vi "load.vi"(8 "error in (no error)":errorcluster, 10 "Node":refnum<k20>, 11 "HP83623A_RF_Generator in":refnum<class "HP83623A_RF_Generator.lvclass">) -> (0 "error out":errorcluster, 2 "node out":refnum<k20>, 3 "HP83623A_RF_Generator out":refnum<class "HP83623A_RF_Generator.lvclass">)   [LabVIEW 2013, in "HP83623A_RF_Generator.lvclass"]
uses:
  HP83623A_RF_Generator.lvclass
  HP83623A.ctl
  HP83623A_RF_Generator.lvclass/HP83623A_RF_Generator.ctl
  <vilib>/xml/Close Reference(Node).vi
  <vilib>/xml/NI_XML.lvlib
  <resource>/objmgr/DOMUserDefRef.rc
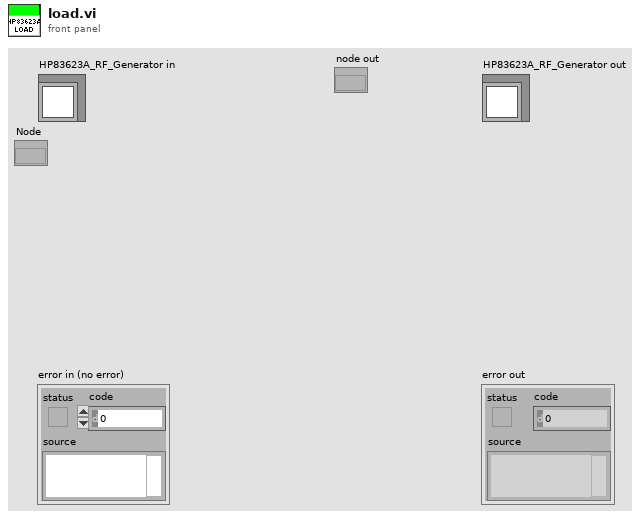
[diagram p1: front panel]
types:
  T1 = typedef "HP83623A_RF_Generator.lvclass/HP83623A.ctl" = cluster{"Frequency (Hz)":dbl, "Power (dBm)":dbl, "Enabled":bool, "initialized":bool, "RF Output On/Off":bool, "External Trigger?":bool, "VISA Session":refnum<visa-resource-name>, "Generator Name":string}
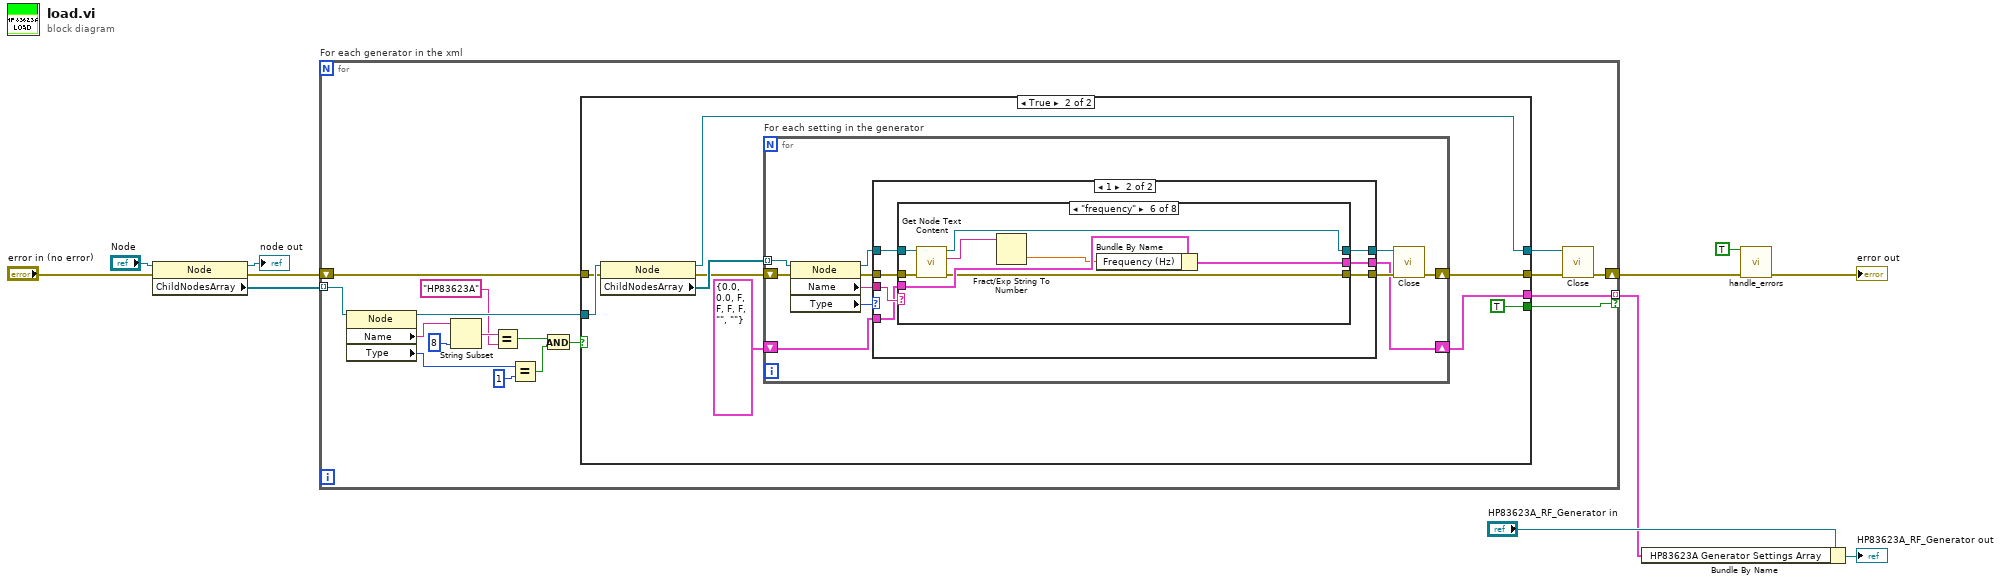
[diagram p0: block diagram]
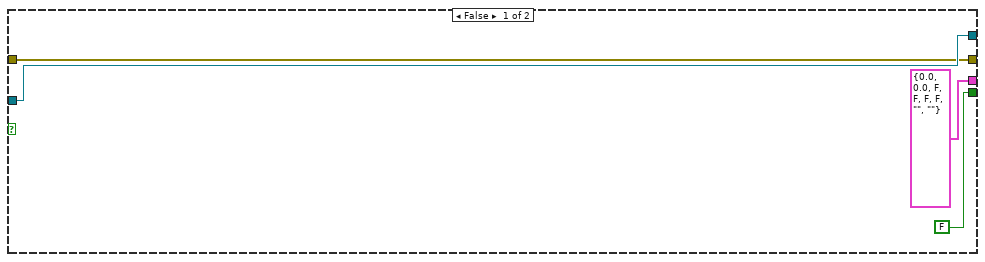
[diagram p2: hidden frame]
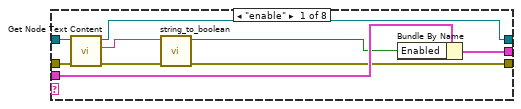
[diagram p4: hidden frame]
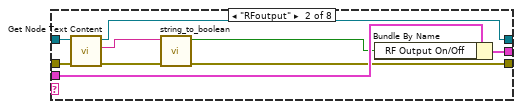
[diagram p5: hidden frame]
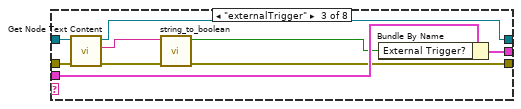
[diagram p6: hidden frame]
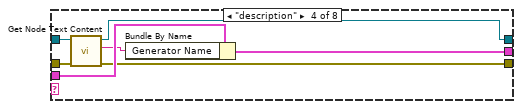
[diagram p7: hidden frame]
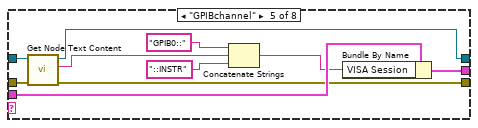
[diagram p8: hidden frame]
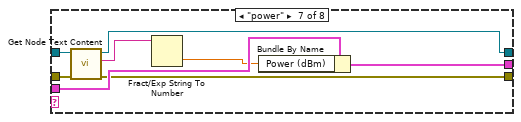
[diagram p9: hidden frame]
diagram:
  n1 = property class="Node"(reference="Node", error in="error in (no error)") -> (reference out=→"node out":refnum<k20>, error out=w4:errorcluster, "ChildNodesArray"=w5:refnum<k20>[])
  n2 = for "For each generator in the xml" {
    tunnel: w5 -> [w23] mode=indexing
    shift-right: [w25] -> w3
    shift-left: w4 -> [w28]
    tunnel: [w12] -> w9 mode=indexing if=w24
    n3 = property class="Node"(reference=w23) -> (reference out=w22:refnum<k20>, "Name"=w18:string, "Type"=w21:i32)  [unwired: 1 in, 1 out]
    n4 = String Subset(string=w18, length (rest)=8 ("length (rest)")) -> (substring=w16:string)  [unwired: 1 in]
    n5 = Equal?(x=w16, y="HP83623A") -> (x = y?=w14:bool)
    n6 = Equal?(x=w21, y=1) -> (x = y?=w19:bool)
    n7 = And(x=w14, y=w19) -> (x .and. y?=w13:bool)
    n8 = case shown="True" w13 {
      tunnel: w22 -> [w32 w41]
      tunnel: w28 -> [w31 w40]
      tunnel: [w32 w37] -> w27
      tunnel: [w31 w36] -> w26
      tunnel: [T1 {"Frequency (Hz)"=0.0, "Power (dBm)"=0.0, "Enabled"=FALSE, "initialized"=FALSE, "RF Output On/Off"=FALSE, "External Trigger?"=FALSE, "VISA Session"="", "Generator Name"=""} ("hp83623a Settings In") w35] -> w12
      tunnel: [FALSE TRUE] -> w24
      frame False {
      }
      frame True {
        n9 = property class="Node"(reference=w41, error in=w40) -> (reference out=w37:refnum<k20>, error out=w38:errorcluster, "ChildNodesArray"=w39:refnum<k20>[])
        n10 = for "For each setting in the generator" {
          shift-right: [w45] -> w36
          shift-left: w38 -> [w49]
          tunnel: w39 -> [w52] mode=indexing
          shift-right: [w43] -> w35
          shift-left: T1 {"Frequency (Hz)"=0.0, "Power (dBm)"=0.0, "Enabled"=FALSE, "initialized"=FALSE, "RF Output On/Off"=FALSE, "External Trigger?"=FALSE, "VISA Session"="", "Generator Name"=""} ("hp83623a Settings In") -> [w44]
          n11 = property class="Node"(reference=w52, error in=w49) -> (reference out=w47:refnum<k20>, error out=w50:errorcluster, "Name"=w51:string, "Type"=w42:i32)
          n12 = case shown="1" w42 {
            tunnel: w51 -> [_ w62]
            tunnel: w50 -> [w54 w61]
            tunnel: [w55 w60] -> w48
            tunnel: w47 -> [w55 w59]
            tunnel: [w54 w58] -> w46
            tunnel: w44 -> [w53 w57]
            tunnel: [w53 w56] -> w43
            frame Default {
            }
            frame 1 {
              n13 = case shown="\"frequency\"" w62 {
                tunnel: w61 -> [w70 w79 w88 w95 w105 w113 w121 w125]
                tunnel: [w63 w72 w81 w90 w101 w109 w117 w125] -> w58
                tunnel: [w67 w76 w85 w91 w102 w110 w118 w124] -> w60
                tunnel: w59 -> [w71 w80 w89 w96 w106 w114 w122 w124]
                tunnel: w57 -> [w69 w78 w87 w94 w104 w112 w120 w123]
                tunnel: [w68 w77 w86 w93 w103 w111 w119 w123] -> w56
                frame "enable" {
                  n14 = call <vilib>:"Get Node Text Content.vi"("error in (no error)"=w70, "node in"=w71) -> ("error out"=w64:errorcluster, "node text"=w66:string, "node out"=w67:refnum<k20>)  [unwired: 7 in]
                  n15 = call "string_to_boolean.vi"("error in"=w64, "string"=w66) -> ("error out"=w63:errorcluster, "boolean"=w65:bool)  [unwired: 8 in]
                  n16 = Bundle By Name(cluster=w69, "Enabled"=w65) -> (w68:T1)
                }
                frame "RFoutput" {
                  n17 = call <vilib>:"Get Node Text Content.vi"("error in (no error)"=w79, "node in"=w80) -> ("error out"=w73:errorcluster, "node text"=w75:string, "node out"=w76:refnum<k20>)  [unwired: 7 in]
                  n18 = call "string_to_boolean.vi"("error in"=w73, "string"=w75) -> ("error out"=w72:errorcluster, "boolean"=w74:bool)  [unwired: 8 in]
                  n19 = Bundle By Name(cluster=w78, "RF Output On/Off"=w74) -> (w77:T1)
                }
                frame "externalTrigger" {
                  n20 = call <vilib>:"Get Node Text Content.vi"("error in (no error)"=w88, "node in"=w89) -> ("error out"=w82:errorcluster, "node text"=w84:string, "node out"=w85:refnum<k20>)  [unwired: 7 in]
                  n21 = call "string_to_boolean.vi"("error in"=w82, "string"=w84) -> ("error out"=w81:errorcluster, "boolean"=w83:bool)  [unwired: 8 in]
                  n22 = Bundle By Name(cluster=w87, "External Trigger?"=w83) -> (w86:T1)
                }
                frame "description" {
                  n23 = call <vilib>:"Get Node Text Content.vi"("error in (no error)"=w95, "node in"=w96) -> ("error out"=w90:errorcluster, "node text"=w92:string, "node out"=w91:refnum<k20>)  [unwired: 7 in]
                  n24 = Bundle By Name(cluster=w94, "Generator Name"=w92) -> (w93:T1)
                }
                frame "GPIBchannel" {
                  n25 = call <vilib>:"Get Node Text Content.vi"("error in (no error)"=w105, "node in"=w106) -> ("error out"=w101:errorcluster, "node text"=w100:string, "node out"=w102:refnum<k20>)  [unwired: 7 in]
                  n26 = Concatenate Strings("GPIB0::" ("string"), w100, "::INSTR" ("string")) -> (w99:string)
                  n27 = Bundle By Name(cluster=w104, "VISA Session"=w99) -> (w103:T1)
                }
                frame "frequency" {
                  n28 = call <vilib>:"Get Node Text Content.vi"("error in (no error)"=w113, "node in"=w114) -> ("error out"=w109:errorcluster, "node text"=w108:string, "node out"=w110:refnum<k20>)  [unwired: 7 in]
                  n29 = Fract/Exp String To Number(string=w108) -> (number=w107:dbl)  [unwired: 3 in, 1 out]
                  n30 = Bundle By Name(cluster=w112, "Frequency (Hz)"=w107) -> (w111:T1)
                }
                frame "power" {
                  n31 = call <vilib>:"Get Node Text Content.vi"("error in (no error)"=w121, "node in"=w122) -> ("error out"=w117:errorcluster, "node text"=w116:string, "node out"=w118:refnum<k20>)  [unwired: 7 in]
                  n32 = Fract/Exp String To Number(string=w116) -> (number=w115:dbl)  [unwired: 3 in, 1 out]
                  n33 = Bundle By Name(cluster=w120, "Power (dBm)"=w115) -> (w119:T1)
                }
                frame Default {
                }
              }
            }
          }
          n34 = call-poly <vilib>:"Close.vi"("error in (no error)"=w46, "node"=w48) -> ("error out"=w45:errorcluster)  [unwired: 7 in]
        }
      }
    }
    n35 = call-poly <vilib>:"Close.vi"("error in (no error)"=w26, "node"=w27) -> ("error out"=w25:errorcluster)  [unwired: 7 in]
  }
  n36 = Bundle By Name(cluster="HP83623A_RF_Generator in", "HP83623A Generator Settings Array"=w9) -> (→"HP83623A_RF_Generator out":refnum<class "HP83623A_RF_Generator.lvclass">)
  n37 = call "handle_errors.vi"("Exit Operation"=TRUE, "error in (no error)"=w3) -> ("error out"=→"error out":errorcluster)  [unwired: 13 in]
